vi "KepcoDCPwr Query Voltage Mode.vi"(0 "VISA Session":refnum<visa-resource-name>, 5 "Model In":string, 7 "Channel Name (\"\")":string, 11 "error in (no error)":errorcluster {"code" format="%.0x"}) -> (4 "VISA Session Out":refnum<visa-resource-name>, 6 "Model Out":string, 8 "channel name out (\"\")":string="\"\"" caption="channel name Out (\"\")", 10 "Mode":string, 14 "Mode (Fixed)":T1(ring), 15 "error out":errorcluster {"code" format="%.0x"})   [LabVIEW 2013]
doc: "This VI reports current state of unit operation.\nStates of operation:\n\nFIXED - unit is outpting a voltage or current \nLIST - The Arb built into the product is executing\nEXT - External analog input is controlling the units output\nGAIN - A portion of external analog inptu is controllong the output\nPROTECT - In BOP 1000 W only, inidcates limit channel supports additional current or voltage\nADDITIVE - The outptu is the sum of a digital value plus the analog reference.\n\n\nNote:\nThis VI is is designed for KLP KLR BIT and BOP 1000 Watt units. Other models report Fixed at all times"
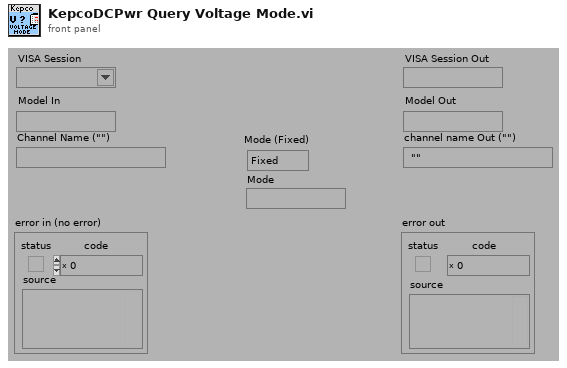
[diagram p1: front panel]
types:
  T1 = enum16{"Fixed", "List", "Transient", "External", "Gain", "Protect"}
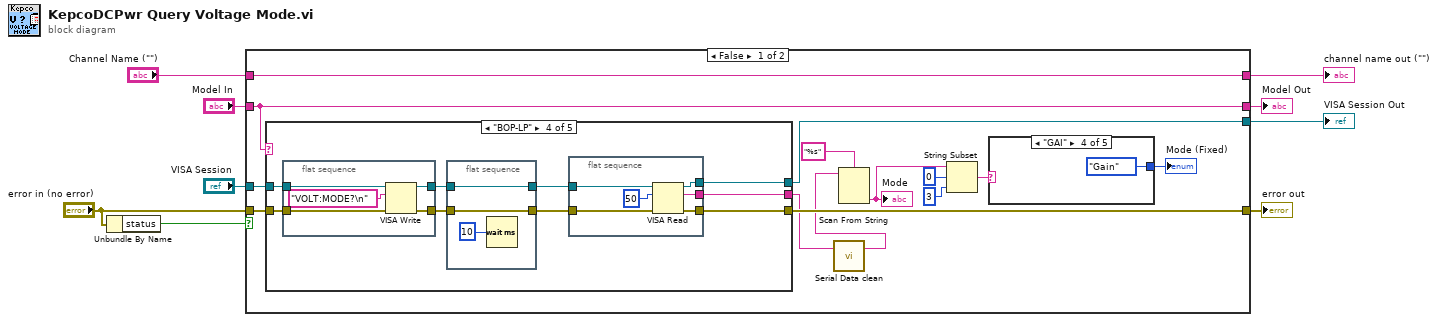
[diagram p0: block diagram]
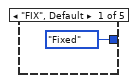
[diagram p2: hidden frame]
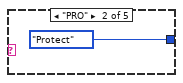
[diagram p3: hidden frame]
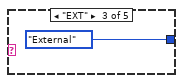
[diagram p4: hidden frame]
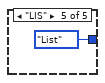
[diagram p5: hidden frame]
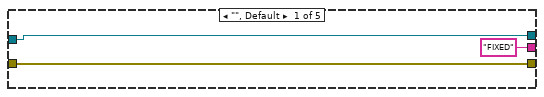
[diagram p6: hidden frame]
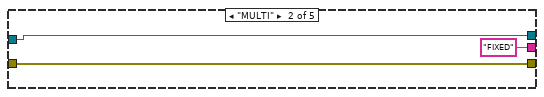
[diagram p7: hidden frame]
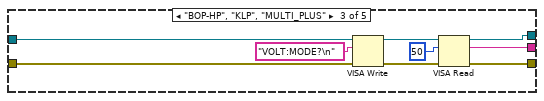
[diagram p8: hidden frame]
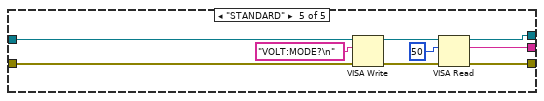
[diagram p9: hidden frame]
diagram:
  n1 = Unbundle By Name("error in (no error)") -> ("status"=w8:bool)
  n2 = case shown="False" w8 {
    tunnel: [w19 w79] -> w9
    tunnel: "error in (no error)" -> [w21 w79]
    tunnel: [w18 w78] -> w6
    tunnel: "VISA Session" -> [w22 w78]
    tunnel: "Model In" -> [w20 w77]
    tunnel: "Channel Name (\"\")" -> [w23 w76]
    tunnel: [w20 w77] -> w2
    tunnel: [w23 w76] -> w1
    frame False {
      n3 = case shown="\"BOP-LP\"" w20 {
        tunnel: w21 -> [w31 w34 w43 w52 w75]
        tunnel: w22 -> [w30 w33 w41 w51 w74]
        tunnel: [w31 w34 w38 w49 w70] -> w19
        tunnel: [w30 w33 w37 w50 w71] -> w18
        tunnel: ["FIXED" ("read buffer") "FIXED" ("read buffer") w35 w48 w67] -> w11
        frame "", Default {
        }
        frame "MULTI" {
        }
        frame "BOP-HP", "KLP", "MULTI_PLUS" {
          n4 = VISA Write(VISA resource name=w41, write buffer="VOLT:MODE?\n", error in (no error)=w43) -> (VISA resource name out=w40:refnum<visa-resource-name>, error out=w42:errorcluster)  [unwired: 1 out]
          n5 = VISA Read(VISA resource name=w40, byte count=u32 50 ("byte count (0)"), error in (no error)=w42) -> (VISA resource name out=w37:refnum<visa-resource-name>, read buffer=w35:string, error out=w38:errorcluster)  [unwired: 1 out]
        }
        frame "BOP-LP" {
          n6 = flat-sequence {
            tunnel: w52 -> [w60]
            tunnel: w51 -> [w59]
            tunnel: [w57] -> w47
            tunnel: [w56] -> w45
            frame #0 {
              n7 = VISA Write(VISA resource name=w59, write buffer="VOLT:MODE?\n", error in (no error)=w60) -> (VISA resource name out=w57:refnum<visa-resource-name>, error out=w56:errorcluster)  [unwired: 1 out]
            }
          }
          n8 = flat-sequence {
            tunnel: w47 -> [w55]
            tunnel: [w55] -> w46
            tunnel: w45 -> [w54]
            tunnel: [w54] -> w44
            frame #0 {
              n9 = Wait (ms)(milliseconds to wait=u32 10 ("byte count (0)")) -> ()  [unwired: 1 out]
            }
          }
          n10 = flat-sequence {
            tunnel: w46 -> [w66]
            tunnel: [w65] -> w50
            tunnel: w44 -> [w64]
            tunnel: [w63] -> w49
            tunnel: [w61] -> w48
            frame #0 {
              n11 = VISA Read(VISA resource name=w66, byte count=u32 50 ("byte count (0)"), error in (no error)=w64) -> (VISA resource name out=w65:refnum<visa-resource-name>, read buffer=w61:string, error out=w63:errorcluster)  [unwired: 1 out]
            }
          }
        }
        frame "STANDARD" {
          n12 = VISA Write(VISA resource name=w74, write buffer="VOLT:MODE?\n", error in (no error)=w75) -> (VISA resource name out=w72:refnum<visa-resource-name>, error out=w69:errorcluster)  [unwired: 1 out]
          n13 = VISA Read(VISA resource name=w72, byte count=u32 50 ("byte count (0)"), error in (no error)=w69) -> (VISA resource name out=w71:refnum<visa-resource-name>, read buffer=w67:string, error out=w70:errorcluster)  [unwired: 1 out]
        }
      }
      n14 = call "Serial Data clean.vi"("string"=w11) -> ("Stripped of Xon Xoff"=w10:string)  [unwired: 2 in]
      n15 = Scan From String(format string="%s", input string=w10) -> (output 1=w15:string)  [unwired: 2 in, 4 out]
      "Mode" <- w15
      n16 = String Subset(string=w15, offset (0)=0, length (rest)=3 ("length (rest)")) -> (substring=w12:string)
      n17 = case shown="\"GAI\"" w12 {
        tunnel: [T1."Fixed" ("Mode (Fixed)") T1."Protect" ("Mode (Fixed)") T1."External" ("Mode (Fixed)") T1."Gain" ("Mode (Fixed)") T1."List" ("Mode (Fixed)")] -> w16
        frame "FIX", Default {
        }
        frame "PRO" {
        }
        frame "EXT" {
        }
        frame "GAI" {
        }
        frame "LIS" {
        }
      }
      "Mode (Fixed)" <- w16
    }
    frame True {
    }
  }
  "error out" <- w9
  "VISA Session Out" <- w6
  "channel name out (\"\")" <- w1
  "Model Out" <- w2
